vi "Periodic Tasks.vi"(8 "error in":errorcluster) -> ()   [LabVIEW 2018]
doc: "This VI runs in parallel to other tasks. It can contain as many user-defined periodic loops as you need. These can carry out PID or other sorts of timed response."
uses:
  <vilib>/Rock Robotics/WPI/Solenoid/WPI_SolenoidValue.ctl
  <vilib>/Rock Robotics/WPI/ThirdParty/Phoenix-LabVIEW/Motor Controller/Controls/CTRE_Phoenix_MotorControl_ControlMode.ctl
  <vilib>/Rock Robotics/WPI/DriverStation/WPI_DriverStationRobotMode2.ctl
  7c96cda5-b0e0-4e2a-8dae-2d02e7ea7fc2.vi
  ca579f97-49ab-43f2-8d57-79325bc44b91.vi
  49744297-d732-4f26-b9df-ea13e04ead65.vi
  0c7d2dc5-c582-4743-8fb3-b9c2bdc871ef.vi
  0ab41fdd-f005-4a41-8abb-d0c1aebc8839.vi
  eb1224c5-d191-4a5a-b208-f0176ff8254b.vi
  4d1e90e2-2e56-4cd0-9c54-8509fccd737b.vi
  fa0b2ed9-014b-4d02-a9e7-965de739ed34.vi
  3bc81077-0bee-49a4-9064-f6dc6ff34700.vi
  c6107473-3bbc-4d68-b130-33bb0f28684e.vi
  bc72f310-a025-467b-8a7d-9af20b832017.vi
  627df16c-e363-45ec-ab0c-cc0e3a3b33f7.vi
  ea05d6e2-4bc2-4863-96e4-0034388c650a.vi
  93672789-ce46-4bc6-a5b5-faff44e817a8.vi
  c8be7294-c6ee-427e-ae78-3199e8744a18.vi
  1c7609ed-6cb5-470b-bbb9-41d14296924d.vi
  50b6936b-a54e-4087-a151-83919d29fb22.vi
  efed0d96-a490-4904-9cbf-ad4873da1ad9.vi
  RobotStates.vi
  Robot Global Data.vi
  <vilib>/Rock Robotics/Network Tables/NT Write Number.vi
  RefNums_DriverStation.vi
  <vilib>/Rock Robotics/WPI/Utilities/WPI_GetSetVariantRefNum.vi
  RefNums_Actuators.vi
  <vilib>/Rock Robotics/WPI/Solenoid/WPI_SolenoidSetEnum.vi
  RefNums_Sensors.vi
  SensorReadings.vi
  Inputs_DriverStation.vi
panel:
  in  "Time in Error Band (ms)":u32=500
  in  "Error Band (in)":dbl=1.0
  in  "Max Down Power":dbl=-0.7 format="%#_13g"
  out "Sensor Loop (ms)":u32
  in  "Enable Plotting":bool
  out "Control Loop Time (ms)":u32
  out "PID Tracking":cluster{"Goal Wheel Position":dbl, dbl}(graph)={"Goal Wheel Position"=0.0, -90.17571233858979}
  out "Contribution Tracking":cluster{dbl, dbl, dbl}(graph)
  in  "N-Int":i32=25
  in  "N-Diff":i32=20
  in  "Kd":dbl=0.01
  in  "Ki":dbl=0.02
  in  "Kp":dbl=0.04
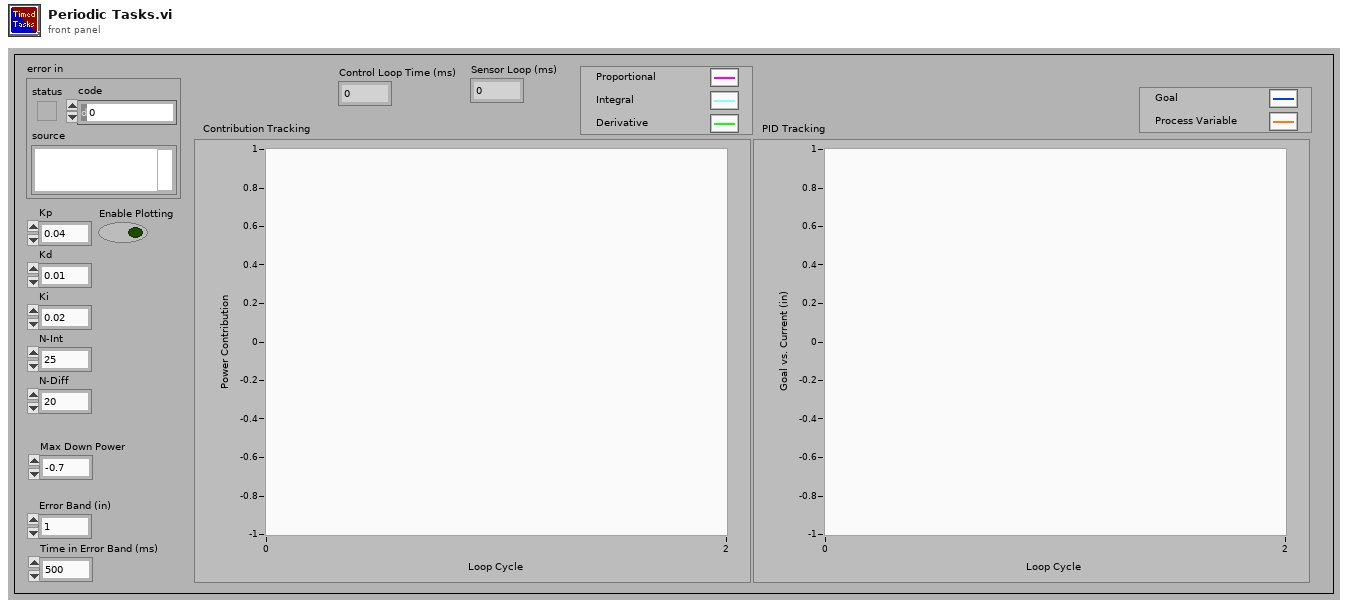
[diagram p1: front panel]
types:
  T1 = typedef "WPI_MotorControlDeviceRef.ctl" = cluster{"DeviceStatus":errorcluster, "Type":T2, "PWM":cluster{"PWM Channel":T3, "DeadBand":T4}, "CAN":cluster{"Device Number":u8, "SetOutput VI Ref":variant, "GetOutput VI Ref":variant, "Enable VI Ref":variant, "Disable VI Ref":variant, "Data":variant}, "Invert":bool, "DIO PWM":cluster{"PWM \"Enable\" Channel":T3, "DIOChannel":T5, "PWM Rate":dbl}}
  T2 = typedef "WPI_MotorControlType.ctl" = enum16{"PWM", "CAN", "DIO PWM"}
  T3 = typedef "FPGA_DIOPWMChannel.ctl" = enum8{"PWM 0", "PWM 1", "PWM 2", "PWM 3", "PWM 4", "PWM 5", "PWM 6", "PWM 7", "PWM 8", "PWM 9", "PWM MXP 0", "PWM MXP 1", "PWM MXP 2", "PWM MXP 3", "PWM MXP 4", "PWM MXP 5", "PWM MXP 6", "PWM MXP 7", "PWM MXP 8", "PWM MXP 9", "Invalid"}
  T4 = typedef "WPI_PWMDeadband.ctl" = cluster{"Name":string, "maxPositivePwm":i32, "minPositivePwm":i32, "centerPwm":i32, "maxNegativePwm":i32, "minNegativePwm":i32, "angularRange":u16}
  T5 = typedef "FPGA_DIOChannel.ctl" = enum8{"DIO 0", "DIO 1", "DIO 2", "DIO 3", "DIO 4", "DIO 5", "DIO 6", "DIO 7", "DIO 8", "DIO 9", "DIO MXP 0", "DIO MXP 1", "DIO MXP 2", "DIO MXP 3", "DIO MXP 4", "DIO MXP 5", "DIO MXP 6", "DIO MXP 7", "DIO MXP 8", "DIO MXP 9", "DIO MXP 10", "DIO MXP 11", "DIO MXP 12", "DIO MXP 13", "DIO MXP 14", "DIO MXP 15", "SPI Port CS1", "SPI Port CS2", "SPI Port CS3", "SPI Port MISO", "SPI Port MOSI", "Invalid"}
  T6 = typedef "WPI_SolenoidDevRef.ctl" = cluster{"DevStatus":errorcluster, "Pneumatics Control Module":u8, "Forward Solenoid Channel":T7, "Reverse Solenoid Channel":T7}
  T7 = typedef "WPI_SolenoidChannel.ctl" = enum8{"Solenoid 0", "Solenoid 1", "Solenoid 2", "Solenoid 3", "Solenoid 4", "Solenoid 5", "Solenoid 6", "Solenoid 7", "Invalid"}
  T8 = typedef "WPI_ServoDeviceRef.ctl" = cluster{"DeviceStatus":errorcluster, "PWM Channel":T3, "DeadBand":T4}
  T9 = typedef "WPI_JoystickDevRef.ctl" = cluster{"Device":T10}
  T10 = typedef "WPI_JoystickDeviceEnum.ctl" = enum16{"USB 0", "USB 1", "USB 2", "USB 3", "USB 4", "USB 5"}
  T11 = typedef "WPI_CompressorDevRef.ctl" = cluster{"DevStatus":errorcluster, "Pneumatics Control Module":u8}
  T12 = typedef "WPI_AccelerometerDevRef.ctl" = cluster{"DevStatus":errorcluster, "Scaling":T13, "Analog Channels":T14, "I2C Bus":T16, "SPI Bus":T17, "Accel Range":T18, "ADXL Axes":T19, "Handle":i32, "Device Address":u8, "Accel Type":enum16{"Analog", "ADXL345 I2C", "ADXL345 SPI", "Internal", "ADXL362 SPI"}}
  T13 = typedef "WPI_AccelerometerScaling.ctl" = cluster{"Gain (VoltsPerG)":dbl, "Center Voltage":dbl}
  T14 = typedef "WPI_AccelerometerAnalogChannels.ctl" = cluster{"X-Axis":T15, "Y-Axis":T15, "Z-Axis":T15}
  T15 = typedef "FPGA_AIChannel.ctl" = enum8{"AI 0", "AI 1", "AI 2", "AI 3", "AI MXP 0", "AI MXP 1", "AI MXP 2", "AI MXP 3", "Invalid"}
  T16 = typedef "i2c_bus.ctl" = enum16{"I2C On-Board", "I2C MXP", "Invalid"}
  T17 = typedef "spi_bus.ctl" = enum16{"SPI On-Board, CS0", "SPI On-Board, CS1", "SPI On-Board, CS2", "SPI On-Board, CS3", "SPI MXP", "Invalid"}
  T18 = typedef "ADXL345 Range.ctl" = u8
  T19 = typedef "WPI_AccelerometerADXL345 Axes.ctl" = cluster{"X-Axis":bool, "Y-Axis":bool, "Z-Axis":bool}
  T20 = typedef "WPI_AnalogChannelDevRef.ctl" = cluster{"DevStatus":errorcluster, "Analog Channel":T15}
  T21 = typedef "WPI_DriverStationRobotMode2.ctl" = enum16{"Autonomous Disabled", "Autonomous Enabled", "Teleop Disabled", "Teleop Enabled", "Disconnected", "Finish", "Test Disabled", "Test Enabled", "Emergency Stopped"}
  T22 = typedef "CTRE_Phoenix_MotorControl_ControlMode.ctl" = u16
  T23 = typedef "WPI_SolenoidValue.ctl" = enum16{"Off", "On", "Forward", "Reverse"}
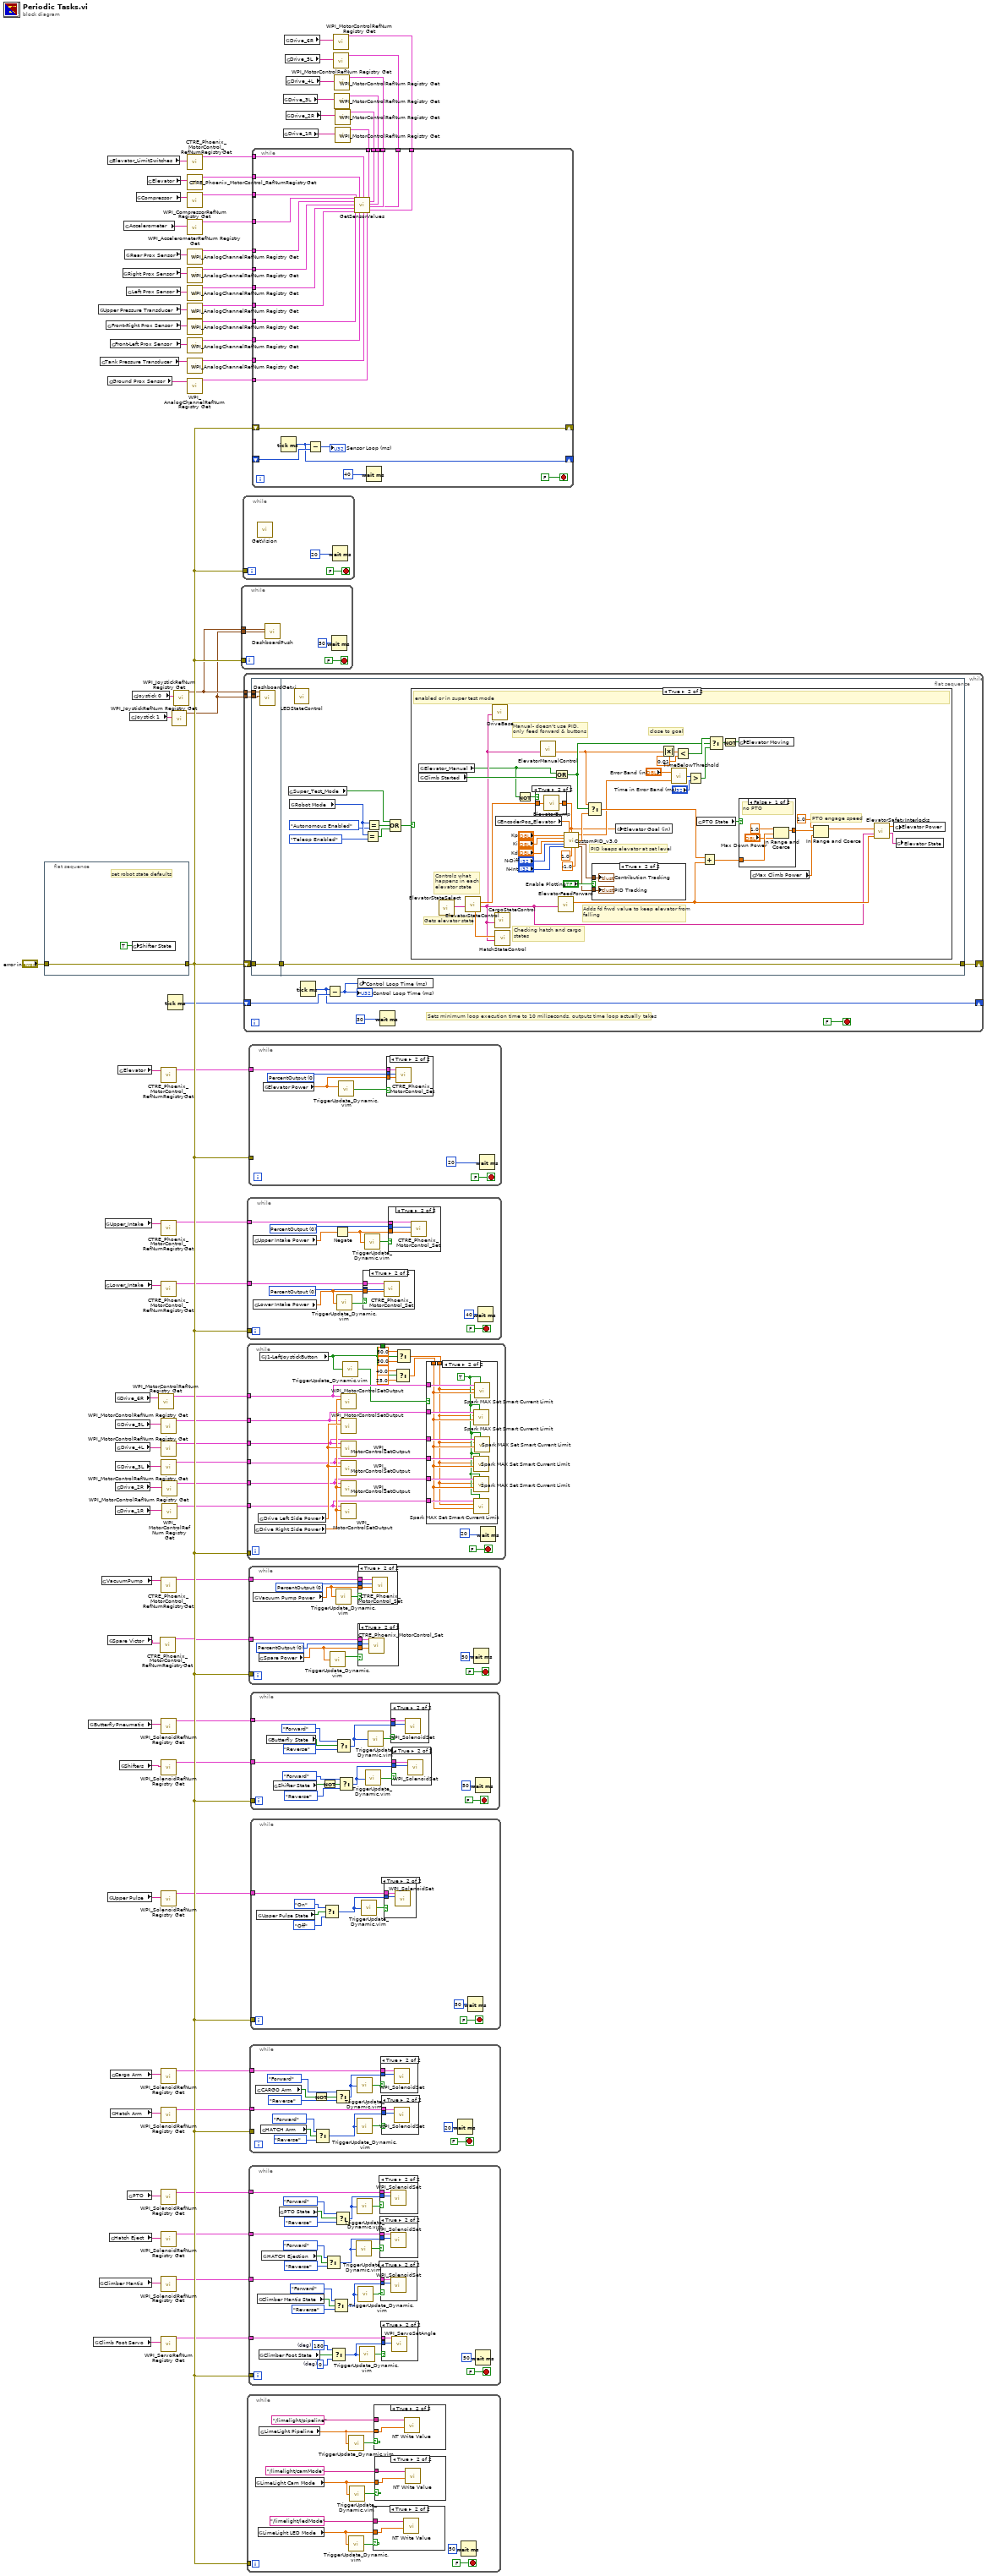
[diagram p0: block diagram]
diagram:
  n1 = flat-sequence {
    tunnel: [w85] -> w83
    tunnel: "error in" -> [w85]
    frame #0 {
      # "set robot state defaults"
      n2 = global write "RobotStates.vi" "Shifter State"(TRUE ("Shifter State")) -> ()
    }
  }
  n3 = global read "RefNums_Actuators.vi" "ButterflyPneumatic"() -> (w80:string)
  n4 = global read "RefNums_Actuators.vi" "Climb Foot Servo"() -> (w17:string)
  n5 = global read "RefNums_Sensors.vi" "Upper Pressure Transducer"() -> (w45:string)
  n6 = global read "RefNums_Actuators.vi" "Climber Mantis"() -> (w60:string)
  n7 = global read "RefNums_Sensors.vi" "Tank Pressure Transducer"() -> (w42:string)
  n8 = global read "RefNums_Actuators.vi" "VacuumPump"() -> (w73:string)
  n9 = global read "RefNums_Actuators.vi" "Upper_Intake"() -> (w70:string)
  n10 = global read "RefNums_Actuators.vi" "Lower_Intake"() -> (w69:string)
  n11 = global read "RefNums_Sensors.vi" "Front-Right Prox Sensor"() -> (w43:string)
  n12 = global read "RefNums_Actuators.vi" "Elevator_LimitSwitches"() -> (w31:string)
  n13 = global read "RefNums_Sensors.vi" "Ground Prox Sensor"() -> (w20:string)
  n14 = global read "RefNums_Actuators.vi" "Spare Victor"() -> (w66:string)
  n15 = global read "RefNums_Actuators.vi" "Upper Pulse"() -> (w76:string)
  n16 = global read "RefNums_Actuators.vi" "Hatch Eject"() -> (w61:string)
  n17 = global read "RefNums_Sensors.vi" "Front-Left Prox Sensor"() -> (w44:string)
  n18 = global read "RefNums_Actuators.vi" "Cargo Arm"() -> (w72:string)
  n19 = global read "RefNums_Actuators.vi" "Hatch Arm"() -> (w62:string)
  n20 = global read "RefNums_Actuators.vi" "Drive_6R"() -> (w14:string)
  n21 = global read "RefNums_Actuators.vi" "Drive_2R"() -> (w10:string)
  n22 = global read "RefNums_Actuators.vi" "Drive_1R"() -> (w15:string)
  n23 = global read "RefNums_Actuators.vi" "Drive_5L"() -> (w13:string)
  n24 = global read "RefNums_Actuators.vi" "Drive_4L"() -> (w12:string)
  n25 = global read "RefNums_Actuators.vi" "Drive_3L"() -> (w11:string)
  n26 = global read "RefNums_Actuators.vi" "Elevator"() -> (w36:string)
  n27 = global read "RefNums_Actuators.vi" "Shifters"() -> (w78:string)
  n28 = global read "RefNums_Sensors.vi" "Right Prox Sensor"() -> (w49:string)
  n29 = global read "RefNums_Sensors.vi" "Accelerometer"() -> (w23:string)
  n30 = global read "RefNums_Sensors.vi" "Rear Prox Sensor"() -> (w51:string)
  n31 = global read "RefNums_Sensors.vi" "Left Prox Sensor"() -> (w50:string)
  n32 = global read "RefNums_Actuators.vi" "PTO"() -> (w64:string)
  n33 = global read "RefNums_DriverStation.vi" "Joystick 1"() -> (w35:string)
  n34 = global read "RefNums_DriverStation.vi" "Joystick 0"() -> (w81:string)
  n35 = global read "RefNums_Actuators.vi" "Compressor"() -> (w55:string)
  n36 = global read "RefNums_Actuators.vi" "Elevator"() -> (w54:string)
  n37 = call <vilib>:"WPI_MotorControlRefNum Registry Get.vi"("refnum name"=w14) -> ("MotorControlDevRef"=w5:T1)  [unwired: 9 in, 1 out]
  n38 = call <vilib>:"CTRE_Phoenix_MotorControl_RefNumRegistryGet.vi"("refnum name"=w66) -> ("PhoenixMotorControlDevRef"=w65:T1)  [unwired: 9 in, 1 out]
  n39 = call <vilib>:"CTRE_Phoenix_MotorControl_RefNumRegistryGet.vi"("refnum name"=w36) -> ("PhoenixMotorControlDevRef"=w82:T1)  [unwired: 9 in, 1 out]
  n40 = call <vilib>:"CTRE_Phoenix_MotorControl_RefNumRegistryGet.vi"("refnum name"=w70) -> ("PhoenixMotorControlDevRef"=w68:T1)  [unwired: 9 in, 1 out]
  n41 = call <vilib>:"CTRE_Phoenix_MotorControl_RefNumRegistryGet.vi"("refnum name"=w69) -> ("PhoenixMotorControlDevRef"=w67:T1)  [unwired: 9 in, 1 out]
  n42 = call <vilib>:"CTRE_Phoenix_MotorControl_RefNumRegistryGet.vi"("refnum name"=w73) -> ("PhoenixMotorControlDevRef"=w74:T1)  [unwired: 9 in, 1 out]
  n43 = call <vilib>:"WPI_SolenoidRefNum Registry Get.vi"("refnum name"=w80) -> ("SolenoidDevRef"=w79:T6)  [unwired: 9 in, 1 out]
  n44 = call <vilib>:"WPI_SolenoidRefNum Registry Get.vi"("refnum name"=w78) -> ("SolenoidDevRef"=w77:T6)  [unwired: 9 in, 1 out]
  n45 = call <vilib>:"WPI_SolenoidRefNum Registry Get.vi"("refnum name"=w76) -> ("SolenoidDevRef"=w75:T6)  [unwired: 9 in, 1 out]
  n46 = call <vilib>:"WPI_SolenoidRefNum Registry Get.vi"("refnum name"=w72) -> ("SolenoidDevRef"=w71:T6)  [unwired: 9 in, 1 out]
  n47 = call <vilib>:"WPI_SolenoidRefNum Registry Get.vi"("refnum name"=w62) -> ("SolenoidDevRef"=w59:T6)  [unwired: 9 in, 1 out]
  n48 = call <vilib>:"WPI_SolenoidRefNum Registry Get.vi"("refnum name"=w64) -> ("SolenoidDevRef"=w63:T6)  [unwired: 9 in, 1 out]
  n49 = call <vilib>:"WPI_SolenoidRefNum Registry Get.vi"("refnum name"=w61) -> ("SolenoidDevRef"=w58:T6)  [unwired: 9 in, 1 out]
  n50 = call <vilib>:"WPI_SolenoidRefNum Registry Get.vi"("refnum name"=w60) -> ("SolenoidDevRef"=w57:T6)  [unwired: 9 in, 1 out]
  n51 = call <vilib>:"WPI_ServoRefNum Registry Get.vi"("refnum name"=w17) -> ("ServoDeviceRef"=w18:T8)  [unwired: 9 in, 1 out]
  n52 = call <vilib>:"WPI_MotorControlRefNum Registry Get.vi"("refnum name"=w13) -> ("MotorControlDevRef"=w6:T1)  [unwired: 9 in, 1 out]
  n53 = call <vilib>:"WPI_MotorControlRefNum Registry Get.vi"("refnum name"=w12) -> ("MotorControlDevRef"=w7:T1)  [unwired: 9 in, 1 out]
  n54 = call <vilib>:"WPI_MotorControlRefNum Registry Get.vi"("refnum name"=w11) -> ("MotorControlDevRef"=w8:T1)  [unwired: 9 in, 1 out]
  n55 = call <vilib>:"WPI_MotorControlRefNum Registry Get.vi"("refnum name"=w10) -> ("MotorControlDevRef"=w9:T1)  [unwired: 9 in, 1 out]
  n56 = call <vilib>:"WPI_MotorControlRefNum Registry Get.vi"("refnum name"=w15) -> ("MotorControlDevRef"=w16:T1)  [unwired: 9 in, 1 out]
  n57 = Tick Count (ms)() -> (millisecond timer value=w56:u32)
  n58 = call <vilib>:"WPI_JoystickRefNum Registry Get.vi"("refnum name"=w35) -> ("JoystickDevRef"=w21:T9)  [unwired: 9 in, 1 out]
  n59 = call <vilib>:"WPI_JoystickRefNum Registry Get.vi"("refnum name"=w81) -> ("JoystickDevRef"=w37:T9)  [unwired: 9 in, 1 out]
  n60 = call <vilib>:"CTRE_Phoenix_MotorControl_RefNumRegistryGet.vi"("refnum name"=w31) -> ("PhoenixMotorControlDevRef"=w30:T1)  [unwired: 9 in, 1 out]
  n61 = call <vilib>:"CTRE_Phoenix_MotorControl_RefNumRegistryGet.vi"("refnum name"=w54) -> ("PhoenixMotorControlDevRef"=w53:T1)  [unwired: 9 in, 1 out]
  n62 = call <vilib>:"WPI_CompressorRefNum Registry Get.vi"("refnum name"=w55) -> ("CompressorDevRef"=w52:T11)  [unwired: 9 in, 1 out]
  n63 = call <vilib>:"WPI_AccelerometerRefNum Registry Get.vi"("refnum name"=w23) -> ("AccelerometerDevRef"=w22:T12)  [unwired: 9 in, 1 out]
  n64 = call <vilib>:"WPI_AnalogChannelRefNum Registry Get.vi"("refnum name"=w51) -> ("AIDeviceRef"=w48:T20)  [unwired: 9 in, 1 out]
  n65 = call <vilib>:"WPI_AnalogChannelRefNum Registry Get.vi"("refnum name"=w49) -> ("AIDeviceRef"=w47:T20)  [unwired: 9 in, 1 out]
  n66 = call <vilib>:"WPI_AnalogChannelRefNum Registry Get.vi"("refnum name"=w50) -> ("AIDeviceRef"=w46:T20)  [unwired: 9 in, 1 out]
  n67 = call <vilib>:"WPI_AnalogChannelRefNum Registry Get.vi"("refnum name"=w45) -> ("AIDeviceRef"=w41:T20)  [unwired: 9 in, 1 out]
  n68 = call <vilib>:"WPI_AnalogChannelRefNum Registry Get.vi"("refnum name"=w43) -> ("AIDeviceRef"=w40:T20)  [unwired: 9 in, 1 out]
  n69 = call <vilib>:"WPI_AnalogChannelRefNum Registry Get.vi"("refnum name"=w44) -> ("AIDeviceRef"=w39:T20)  [unwired: 9 in, 1 out]
  n70 = call <vilib>:"WPI_AnalogChannelRefNum Registry Get.vi"("refnum name"=w42) -> ("AIDeviceRef"=w38:T20)  [unwired: 9 in, 1 out]
  n71 = call <vilib>:"WPI_AnalogChannelRefNum Registry Get.vi"("refnum name"=w20) -> ("AIDeviceRef"=w19:T20)  [unwired: 9 in, 1 out]
  n72 = while {
    tunnel: w37 -> [w88]
    tunnel: w83 -> [_]
    tunnel: w21 -> [w86]
    stop <- FALSE stop-if-true
    n73 = call "DashboardPush.vi"("Joystick 0 Ref"=w88, "Joystick 1 Ref"=w86) -> ()  [unwired: 14 in]
    n74 = Wait (ms)(milliseconds to wait=u32 50) -> ()  [unwired: 1 out]
  }
  n75 = while {
    tunnel: w83 -> [_]
    stop <- FALSE stop-if-true
    n76 = call "GetVision.vi"() -> ()  [unwired: 12 in]
    n77 = Wait (ms)(milliseconds to wait=u32 20) -> ()  [unwired: 1 out]
  }
  n78 = while {
    shift-right: [w98] -> _
    shift-left: w83 -> [w100]
    tunnel: w37 -> [w97]
    shift-right: [w95] -> _
    shift-left: w56 -> [w96]
    tunnel: w21 -> [w93]
    stop <- FALSE stop-if-true
    # "Sets minimum loop execution time to 10 miliseconds, outputs time loop actually takes"
    n79 = flat-sequence {
      tunnel: w97 -> [w104]
      tunnel: w100 -> [w103]
      tunnel: [w103] -> w99
      tunnel: w93 -> [w102]
      tunnel: w99 -> [w112]
      tunnel: [w112] -> w98
      frame #0 {
        n80 = call "DashboardGetvi.vi"("Joystick 2"=w102, "Joystick 1"=w104) -> ()  [unwired: 8 in]
      }
      frame #1 {
        n81 = global read "Inputs_DriverStation.vi" "Super_Test_Mode"() -> (w105:bool)
        n82 = global read "Robot Global Data.vi" "Robot Mode"() -> (w109:T21)
        n83 = call "LEDStateControl.vi"() -> ()  [unwired: 12 in]
        n84 = Equal?(x=w109, y=WPI_DriverStationRobotMode2."Teleop Enabled") -> (x = y?=w110:bool)
        n85 = Equal?(x=w109, y=WPI_DriverStationRobotMode2."Autonomous Enabled") -> (x = y?=w111:bool)
        n86 = Compound Arithmetic op=OR(w105, w111, w110) -> (w106:bool)
        n87 = case shown="True" w106 {
          frame False {
            # "disabled and not in super test mode"
          }
          frame True {
            # "PTO engage speed"
            # "close to goal"
            # "PID keeps elevator at set level"
            # "Manual- doesn't use PID,\nonly feed forward & buttons"
            # "Adds fd frwd value to keep elevator from falling"
            # "Checking hatch and cargo \nstates"
            # "Controls what\nhappens in each \nelevator state"
            # "Gets elevator state"
            # "enabled or in super test mode"
            n88 = global read "Inputs_DriverStation.vi" "Elevator_Manual"() -> (w113:bool)
            n89 = global read "RobotStates.vi" "Climb Started"() -> (w138:bool)
            n90 = call "ElevatorStateSelect.vi"() -> ("Elevator State"=w151:string)  [unwired: 11 in]
            n91 = call "ElevatorStateControl.vi"("Elevator State"=w151) -> ("Elevator State Out"=w121:string, "Target Elevator Position"=w154:dbl, "Target Vacuum Pump Power"=w139:dbl)  [unwired: 8 in]
            n92 = call "DriveBase.vi"("Elevator State"=w121) -> ()  [unwired: 11 in]
            n93 = call "CargoStateControl.vi"("Elevator State"=w121) -> ()  [unwired: 11 in]
            n94 = call "HatchStateControl.vi"("Elevator State"=w121, "Vacuum Pump Power"=w139) -> ()  [unwired: 10 in]
            n95 = global read "SensorReadings.vi" "EncoderPos_Elevator"() -> (w149:dbl)
            n96 = Not(x=w113) -> (.not. x?=w114:bool)
            n97 = case shown="True" w114 {
              tunnel: w154 -> [w155 w157]
              tunnel: [w155 w156] -> w115
              frame False {
              }
              frame True {
                n98 = call "ElevatorBump.vi"("Elevator Goal In (in)"=w157) -> ("Elevator Goal Out (in)"=w156:dbl)
              }
            }
            n99 = call "ElevatorManualControl.vi"("Elevator State"=w121) -> ("Manual Contribution"=w122:dbl)  [unwired: 10 in]
            n100 = Or(x=w113, y=w138) -> (x .or. y?=w124:bool)
            n101 = call "ElevatorFeedForward.vi"("Elevator State"=w121) -> ("Feed Forward Contribution"=w135:dbl)  [unwired: 10 in]
            n102 = call "CustomPID_v3.0.vi"("Kp"="Kp", "Process Variable"=w149, "Goal"=w115, "Ki"="Ki", "Kd"="Kd", "N-Diff"="N-Diff", "N-Int"="N-Int", "Max Ouput"=1.0, "Min Output"=-1.0) -> ("Current Error"=w130:dbl, "Command"=w150:dbl, "Contribution Tracking"=w141:cluster{dbl, dbl, dbl}, "PID Tracking"=w140:cluster{"Goal Wheel Position":dbl, dbl})  [unwired: 3 in]
            n103 = Select(t=w122, s=w124, f=w150) -> (s? t:f=w152:dbl)
            n104 = case shown="True" "Enable Plotting" {
              tunnel: w141 -> [_ w167]
              tunnel: w140 -> [_ w166]
              frame False {
              }
              frame True {
                "Contribution Tracking" <- w167
                "PID Tracking" <- w166
              }
            }
            n105 = global write "RobotStates.vi" "Elevator Goal (in)"(w115) -> ()
            n106 = Absolute Value(x=w122) -> (abs(x)=w129:dbl)
            n107 = call "TimeBelowThreshold.vi"("Current Value"=w130, "Threshold"="Error Band (in)") -> ("Time Below"=w132:u32)  [unwired: 3 in]
            n108 = Less?(x=w129, y=0.01) -> (x < y?=w128:bool)
            n109 = Greater?(x=w132, y="Time in Error Band (ms)") -> (0:w123:bool)
            n110 = global read "RobotStates.vi" "PTO State"() -> (w120:bool)
            n111 = Add(x=w152, y=w135) -> (x+y=w134:dbl)
            n112 = Select(t=w128, s=w124, f=w123) -> (s? t:f=w127:bool)
            n113 = Not(x=w127) -> (.not. x?=w126:bool)
            n114 = global write "RobotStates.vi" "Elevator Moving"(w126) -> ()
            n115 = case shown="False" w120 {
              tunnel: w134 -> [w161 w164]
              tunnel: [w158 w165] -> w118
              frame False {
                # "no PTO"
                n116 = In Range and Coerce(upper limit=1.0, x=w161, lower limit="Max Down Power") -> (coerced(x)=w158:dbl)  [unwired: 1 out]
              }
              frame True {
                # "PTO"
                n117 = In Range and Coerce(upper limit=1.0, x=w164, lower limit=-1.0) -> (coerced(x)=w165:dbl)  [unwired: 1 out]
              }
            }
            n118 = global read "RobotStates.vi" "Max Climb Power"() -> (w116:dbl)
            n119 = In Range and Coerce(upper limit=1.0, x=w118, lower limit=w116) -> (coerced(x)=w119:dbl)  [unwired: 1 out]
            n120 = call "ElevatorSafetyInterlocks.vi"("Feed Forward Contribution"=w135, "Elevator State In"=w121, "Elevator Power In"=w119) -> ("Elevator State Out"=w136:string, "Elevator Power Out"=w137:dbl)  [unwired: 7 in]
            n121 = global write "RobotStates.vi" "Elevator Power"(w137) -> ()
            n122 = global write "RobotStates.vi" "Elevator State"(w136) -> ()
          }
        }
      }
    }
    n123 = Tick Count (ms)() -> (millisecond timer value=w95:u32)
    n124 = Subtract(x=w95, y=w96) -> (x-y=w94:u32)
    "Control Loop Time (ms)" <- w94
    n125 = global write "SensorReadings.vi" "Control Loop Time (ms)"(w94) -> ()
    n126 = Wait (ms)(milliseconds to wait=u32 30) -> ()  [unwired: 1 out]
  }
  n127 = while {
    tunnel: w83 -> [_]
    tunnel: w16 -> [w181]
    tunnel: w9 -> [w180]
    tunnel: w8 -> [w179]
    tunnel: w7 -> [w178]
    tunnel: w6 -> [w177]
    tunnel: w5 -> [w176]
    tunnel: [w168] -> _
    stop <- FALSE stop-if-true
    n128 = global read "RobotStates.vi" "Drive Right Side Power"() -> (w182:dbl)
    n129 = global read "RobotStates.vi" "Drive Left Side Power"() -> (w183:dbl)
    n130 = global read "Inputs_DriverStation.vi" "J1-LeftJoystickButton"() -> (w168:bool)
    n131 = call <vilib>:"WPI_MotorControlSetOutput.vi"("Output"=w182, "MotorControlDevRef"=w176) -> ()  [unwired: 7 in, 3 out]
    n132 = call <vilib>:"WPI_MotorControlSetOutput.vi"("Output"=w183, "MotorControlDevRef"=w177) -> ()  [unwired: 7 in, 3 out]
    n133 = call <vilib>:"WPI_MotorControlSetOutput.vi"("Output"=w183, "MotorControlDevRef"=w178) -> ()  [unwired: 7 in, 3 out]
    n134 = call <vilib>:"WPI_MotorControlSetOutput.vi"("Output"=w183, "MotorControlDevRef"=w179) -> ()  [unwired: 7 in, 3 out]
    n135 = call <vilib>:"WPI_MotorControlSetOutput.vi"("Output"=w182, "MotorControlDevRef"=w180) -> ()  [unwired: 7 in, 3 out]
    n136 = call <vilib>:"WPI_MotorControlSetOutput.vi"("Output"=w182, "MotorControlDevRef"=w181) -> ()  [unwired: 7 in, 3 out]
    n137 = call "TriggerUpdate_Dynamic.vim"("Trigger"=w168) -> ("Update"=w169:bool)
    n138 = Select(t=40.0, s=w168, f=25.0 ("Free Speed Current Limit (20A)")) -> (s? t:f=w174:dbl)
    n139 = Select(t=80.0, s=w168, f=50.0 ("Free Speed Current Limit (20A)")) -> (s? t:f=w170:dbl)
    n140 = case shown="True" w169 {
      tunnel: w181 -> [_ w194]
      tunnel: w180 -> [_ w193]
      tunnel: w179 -> [_ w192]
      tunnel: w178 -> [_ w191]
      tunnel: w177 -> [_ w190]
      tunnel: w176 -> [_ w189]
      tunnel: w174 -> [_ w188]
      tunnel: w170 -> [_ w186]
      frame False {
      }
      frame True {
        w187 = TRUE
        n141 = call <vilib>:"Spark MAX Set Smart Current Limit.vi"("Linearized Limit Enabled (F)"=w187, "Free Speed Current Limit (20A)"=w188, "Primay Current Limit (80A)"=w186, "MotorControlDeviceRef in"=w192) -> ()  [unwired: 6 in, 2 out]
        n142 = call <vilib>:"Spark MAX Set Smart Current Limit.vi"("Linearized Limit Enabled (F)"=w187, "Free Speed Current Limit (20A)"=w188, "Primay Current Limit (80A)"=w186, "MotorControlDeviceRef in"=w190) -> ()  [unwired: 6 in, 2 out]
        n143 = call <vilib>:"Spark MAX Set Smart Current Limit.vi"("Linearized Limit Enabled (F)"=w187, "Free Speed Current Limit (20A)"=w188, "Primay Current Limit (80A)"=w186, "MotorControlDeviceRef in"=w193) -> ()  [unwired: 6 in, 2 out]
        n144 = call <vilib>:"Spark MAX Set Smart Current Limit.vi"("Linearized Limit Enabled (F)"=w187, "Free Speed Current Limit (20A)"=w188, "Primay Current Limit (80A)"=w186, "MotorControlDeviceRef in"=w194) -> ()  [unwired: 6 in, 2 out]
        n145 = call <vilib>:"Spark MAX Set Smart Current Limit.vi"("Linearized Limit Enabled (F)"=w187, "Free Speed Current Limit (20A)"=w188, "Primay Current Limit (80A)"=w186, "MotorControlDeviceRef in"=w189) -> ()  [unwired: 6 in, 2 out]
        n146 = call <vilib>:"Spark MAX Set Smart Current Limit.vi"("Linearized Limit Enabled (F)"=w187, "Free Speed Current Limit (20A)"=w188, "Primay Current Limit (80A)"=w186, "MotorControlDeviceRef in"=w191) -> ()  [unwired: 6 in, 2 out]
      }
    }
    n147 = Wait (ms)(milliseconds to wait=u32 20) -> ()  [unwired: 1 out]
  }
  n148 = while {
    tunnel: w83 -> [_]
    stop <- FALSE stop-if-true
    n149 = global read "RobotStates.vi" "LimeLight Cam Mode"() -> (w198:dbl)
    n150 = global read "RobotStates.vi" "LimeLight LED Mode"() -> (w201:dbl)
    n151 = global read "RobotStates.vi" "LimeLight Pipeline"() -> (w195:dbl)
    n152 = call "TriggerUpdate_Dynamic.vim"("Trigger"=w201) -> ("Update"=w203:bool)
    n153 = call "TriggerUpdate_Dynamic.vim"("Trigger"=w195) -> ("Update"=w197:bool)
    n154 = call "TriggerUpdate_Dynamic.vim"("Trigger"=w198) -> ("Update"=w200:bool)
    n155 = case shown="True" w203 {
      tunnel: "/limelight/ledMode" ("Name") -> [_ w211]
      tunnel: w201 -> [_ w210]
      frame False {
      }
      frame True {
        n156 = call-poly <vilib>:"NT Write Value.vi"("Numeric"=w210, "Name"=w211) -> ()  [unwired: 9 in, 1 out]
      }
    }
    n157 = case shown="True" w197 {
      tunnel: "/limelight/pipeline" ("Name") -> [_ w207]
      tunnel: w195 -> [_ w206]
      frame False {
      }
      frame True {
        n158 = call-poly <vilib>:"NT Write Value.vi"("Numeric"=w206, "Name"=w207) -> ()  [unwired: 9 in, 1 out]
      }
    }
    n159 = case shown="True" w200 {
      tunnel: "/limelight/camMode" ("Name") -> [_ w209]
      tunnel: w198 -> [_ w208]
      frame False {
      }
      frame True {
        n160 = call-poly <vilib>:"NT Write Value.vi"("Numeric"=w208, "Name"=w209) -> ()  [unwired: 9 in, 1 out]
      }
    }
    n161 = Wait (ms)(milliseconds to wait=u32 50) -> ()  [unwired: 1 out]
  }
  n162 = while {
    tunnel: w68 -> [w222]
    tunnel: w67 -> [w221]
    tunnel: w83 -> [_]
    stop <- FALSE stop-if-true
    w219 = T22 0 items=["PercentOutput"=0, "Position"=1, "Velocity"=2, "Current"=3, "Follower"=5, "MotionProfile"=6, "MotionMagic"=7, "MotionProfileArc"=10, "Disabled"=15] ("Control Mode")
    w220 = T22 0 items=["PercentOutput"=0, "Position"=1, "Velocity"=2, "Current"=3, "Follower"=5, "MotionProfile"=6, "MotionMagic"=7, "MotionProfileArc"=10, "Disabled"=15] ("Control Mode")
    n163 = global read "RobotStates.vi" "Upper Intake Power"() -> (w216:dbl)
    n164 = global read "RobotStates.vi" "Lower Intake Power"() -> (w214:dbl)
    n165 = Negate(x=w216) -> (-x=w212:dbl)
    n166 = call "TriggerUpdate_Dynamic.vim"("Trigger"=w214) -> ("Update"=w213:bool)
    n167 = case shown="True" w213 {
      tunnel: w221 -> [_ w225]
      tunnel: w219 -> [_ w224]
      tunnel: w214 -> [_ w223]
      frame False {
      }
      frame True {
        n168 = call <vilib>:"CTRE_Phoenix_MotorControl_Set.vi"("Output"=w223, "Control Mode"=w224, "PhoenixMotorControlDevRef"=w225) -> ()  [unwired: 7 in, 2 out]
      }
    }
    n169 = call "TriggerUpdate_Dynamic.vim"("Trigger"=w212) -> ("Update"=w215:bool)
    n170 = case shown="True" w215 {
      tunnel: w222 -> [_ w228]
      tunnel: w220 -> [_ w227]
      tunnel: w212 -> [_ w226]
      frame False {
      }
      frame True {
        n171 = call <vilib>:"CTRE_Phoenix_MotorControl_Set.vi"("Output"=w226, "Control Mode"=w227, "PhoenixMotorControlDevRef"=w228) -> ()  [unwired: 7 in, 2 out]
      }
    }
    n172 = Wait (ms)(milliseconds to wait=u32 40) -> ()  [unwired: 1 out]
  }
  n173 = while {
    tunnel: w83 -> [_]
    tunnel: w82 -> [w233]
    stop <- FALSE stop-if-true
    w232 = T22 0 items=["PercentOutput"=0, "Position"=1, "Velocity"=2, "Current"=3, "Follower"=5, "MotionProfile"=6, "MotionMagic"=7, "MotionProfileArc"=10, "Disabled"=15] ("Control Mode")
    n174 = global read "RobotStates.vi" "Elevator Power"() -> (w231:dbl)
    n175 = call "TriggerUpdate_Dynamic.vim"("Trigger"=w231) -> ("Update"=w230:bool)
    n176 = case shown="True" w230 {
      tunnel: w233 -> [_ w237]
      tunnel: w232 -> [_ w236]
      tunnel: w231 -> [_ w235]
      frame False {
      }
      frame True {
        n177 = call <vilib>:"CTRE_Phoenix_MotorControl_Set.vi"("Output"=w235, "Control Mode"=w236, "PhoenixMotorControlDevRef"=w237) -> ()  [unwired: 7 in, 2 out]
      }
    }
    n178 = Wait (ms)(milliseconds to wait=u32 20) -> ()  [unwired: 1 out]
  }
  n179 = while {
    tunnel: w74 -> [w247]
    tunnel: w65 -> [w246]
    tunnel: w83 -> [_]
    stop <- FALSE stop-if-true
    w238 = T22 0 items=["PercentOutput"=0, "Position"=1, "Velocity"=2, "Current"=3, "Follower"=5, "MotionProfile"=6, "MotionMagic"=7, "MotionProfileArc"=10, "Disabled"=15] ("Control Mode")
    w245 = T22 0 items=["PercentOutput"=0, "Position"=1, "Velocity"=2, "Current"=3, "Follower"=5, "MotionProfile"=6, "MotionMagic"=7, "MotionProfileArc"=10, "Disabled"=15] ("Control Mode")
    n180 = global read "RobotStates.vi" "Vacuum Pump Power"() -> (w242:dbl)
    n181 = global read "RobotStates.vi" "Spare Power"() -> (w240:dbl)
    n182 = call "TriggerUpdate_Dynamic.vim"("Trigger"=w240) -> ("Update"=w239:bool)
    n183 = call "TriggerUpdate_Dynamic.vim"("Trigger"=w242) -> ("Update"=w241:bool)
    n184 = case shown="True" w241 {
      tunnel: w247 -> [_ w253]
      tunnel: w245 -> [_ w252]
      tunnel: w242 -> [_ w251]
      frame False {
      }
      frame True {
        n185 = call <vilib>:"CTRE_Phoenix_MotorControl_Set.vi"("Output"=w251, "Control Mode"=w252, "PhoenixMotorControlDevRef"=w253) -> ()  [unwired: 7 in, 2 out]
      }
    }
    n186 = case shown="True" w239 {
      tunnel: w246 -> [_ w250]
      tunnel: w238 -> [_ w249]
      tunnel: w240 -> [_ w248]
      frame False {
      }
      frame True {
        n187 = call <vilib>:"CTRE_Phoenix_MotorControl_Set.vi"("Output"=w248, "Control Mode"=w249, "PhoenixMotorControlDevRef"=w250) -> ()  [unwired: 7 in, 2 out]
      }
    }
    n188 = Wait (ms)(milliseconds to wait=u32 50) -> ()  [unwired: 1 out]
  }
  n189 = while {
    tunnel: w63 -> [w279]
    tunnel: w58 -> [w278]
    tunnel: w57 -> [w277]
    tunnel: w83 -> [_]
    tunnel: w18 -> [w258]
    stop <- FALSE stop-if-true
    w255 = 180  # (deg)
    w257 = 0  # (deg)
    n190 = global read "RobotStates.vi" "Climber Mantis State"() -> (w272:bool)
    n191 = global read "RobotStates.vi" "Climber Foot State"() -> (w254:bool)
    n192 = global read "RobotStates.vi" "HATCH Ejection"() -> (w274:bool)
    n193 = global read "RobotStates.vi" "PTO State"() -> (w260:bool)
    n194 = Select(t=WPI_SolenoidValue."Forward" ("Value"), s=w274, f=WPI_SolenoidValue."Reverse") -> (s? t:f=w264:T23)
    n195 = Select(t=w255, s=w254, f=w257) -> (s? t:f=w256:i32)
    n196 = Select(t=WPI_SolenoidValue."Forward" ("Value"), s=w272, f=WPI_SolenoidValue."Reverse") -> (s? t:f=w262:T23)
    n197 = Select(t=WPI_SolenoidValue."Forward" ("Value"), s=w260, f=WPI_SolenoidValue."Reverse") -> (s? t:f=w266:T23)
    n198 = call "TriggerUpdate_Dynamic.vim"("Trigger"=w264) -> ("Update"=w263:bool)
    n199 = call "TriggerUpdate_Dynamic.vim"("Trigger"=w266) -> ("Update"=w265:bool)
    n200 = call "TriggerUpdate_Dynamic.vim"("Trigger"=w262) -> ("Update"=w261:bool)
    n201 = call "TriggerUpdate_Dynamic.vim"("Trigger"=w256) -> ("Update"=w259:bool)
    n202 = case shown="True" w265 {
      tunnel: w279 -> [_ w287]
      tunnel: w266 -> [_ w286]
      frame False {
      }
      frame True {
        n203 = call-poly <vilib>:"WPI_SolenoidSet.vi"("Value"=w286, "SolenoidDevRef"=w287) -> ()  [unwired: 8 in, 2 out]
      }
    }
    n204 = case shown="True" w263 {
      tunnel: w278 -> [_ w285]
      tunnel: w264 -> [_ w284]
      frame False {
      }
      frame True {
        n205 = call-poly <vilib>:"WPI_SolenoidSet.vi"("Value"=w284, "SolenoidDevRef"=w285) -> ()  [unwired: 8 in, 2 out]
      }
    }
    n206 = case shown="True" w261 {
      tunnel: w277 -> [_ w283]
      tunnel: w262 -> [_ w282]
      frame False {
      }
      frame True {
        n207 = call-poly <vilib>:"WPI_SolenoidSet.vi"("Value"=w282, "SolenoidDevRef"=w283) -> ()  [unwired: 8 in, 2 out]
      }
    }
    n208 = case shown="True" w259 {
      tunnel: w256 -> [_ w280]
      tunnel: w258 -> [_ w281]
      frame False {
      }
      frame True {
        n209 = call <vilib>:"WPI_ServoSetAngle.vi"("Angle"=w280, "ServoDeviceRef"=w281) -> ()  [unwired: 8 in, 2 out]
      }
    }
    n210 = Wait (ms)(milliseconds to wait=u32 50) -> ()  [unwired: 1 out]
  }
  n211 = while {
    tunnel: w71 -> [w302]
    tunnel: w59 -> [w301]
    tunnel: w83 -> [_]
    stop <- FALSE stop-if-true
    n212 = global read "RobotStates.vi" "CARGO Arm"() -> (w300:bool)
    n213 = global read "RobotStates.vi" "HATCH Arm"() -> (w297:bool)
    n214 = Not(x=w300) -> (.not. x?=w288:bool)
    n215 = Select(t=WPI_SolenoidValue."Forward" ("Value"), s=w297, f=WPI_SolenoidValue."Reverse") -> (s? t:f=w290:T23)
    n216 = Select(t=WPI_SolenoidValue."Forward" ("Value"), s=w288, f=WPI_SolenoidValue."Reverse") -> (s? t:f=w292:T23)
    n217 = call "TriggerUpdate_Dynamic.vim"("Trigger"=w292) -> ("Update"=w291:bool)
    n218 = call "TriggerUpdate_Dynamic.vim"("Trigger"=w290) -> ("Update"=w289:bool)
    n219 = case shown="True" w291 {
      tunnel: w302 -> [_ w306]
      tunnel: w292 -> [_ w305]
      frame False {
      }
      frame True {
        n220 = call-poly <vilib>:"WPI_SolenoidSet.vi"("Value"=w305, "SolenoidDevRef"=w306) -> ()  [unwired: 8 in, 2 out]
      }
    }
    n221 = case shown="True" w289 {
      tunnel: w301 -> [_ w304]
      tunnel: w290 -> [_ w303]
      frame False {
      }
      frame True {
        n222 = call-poly <vilib>:"WPI_SolenoidSet.vi"("Value"=w303, "SolenoidDevRef"=w304) -> ()  [unwired: 8 in, 2 out]
      }
    }
    n223 = Wait (ms)(milliseconds to wait=u32 20) -> ()  [unwired: 1 out]
  }
  n224 = while {
    tunnel: w79 -> [w321]
    tunnel: w77 -> [w320]
    tunnel: w83 -> [_]
    stop <- FALSE stop-if-true
    n225 = global read "RobotStates.vi" "Butterfly State"() -> (w317:bool)
    n226 = global read "RobotStates.vi" "Shifter State"() -> (w316:bool)
    n227 = Not(x=w316) -> (.not. x?=w307:bool)
    n228 = Select(t=WPI_SolenoidValue."Forward" ("Value"), s=w317, f=WPI_SolenoidValue."Reverse") -> (s? t:f=w311:T23)
    n229 = Select(t=WPI_SolenoidValue."Forward" ("Value"), s=w307, f=WPI_SolenoidValue."Reverse") -> (s? t:f=w309:T23)
    n230 = call "TriggerUpdate_Dynamic.vim"("Trigger"=w309) -> ("Update"=w308:bool)
    n231 = call "TriggerUpdate_Dynamic.vim"("Trigger"=w311) -> ("Update"=w310:bool)
    n232 = case shown="True" w310 {
      tunnel: w321 -> [_ w325]
      tunnel: w311 -> [_ w324]
      frame False {
      }
      frame True {
        n233 = call-poly <vilib>:"WPI_SolenoidSet.vi"("Value"=w324, "SolenoidDevRef"=w325) -> ()  [unwired: 8 in, 2 out]
      }
    }
    n234 = case shown="True" w308 {
      tunnel: w320 -> [_ w323]
      tunnel: w309 -> [_ w322]
      frame False {
      }
      frame True {
        n235 = call-poly <vilib>:"WPI_SolenoidSet.vi"("Value"=w322, "SolenoidDevRef"=w323) -> ()  [unwired: 8 in, 2 out]
      }
    }
    n236 = Wait (ms)(milliseconds to wait=u32 50) -> ()  [unwired: 1 out]
  }
  n237 = while {
    tunnel: w75 -> [w333]
    tunnel: w83 -> [_]
    stop <- FALSE stop-if-true
    n238 = global read "RobotStates.vi" "Upper Pulse State"() -> (w332:bool)
    n239 = Select(t=WPI_SolenoidValue."On" ("Value"), s=w332, f=WPI_SolenoidValue."Off") -> (s? t:f=w327:T23)
    n240 = call "TriggerUpdate_Dynamic.vim"("Trigger"=w327) -> ("Update"=w326:bool)
    n241 = case shown="True" w326 {
      tunnel: w333 -> [_ w335]
      tunnel: w327 -> [_ w334]
      frame False {
      }
      frame True {
        n242 = call-poly <vilib>:"WPI_SolenoidSet.vi"("Value"=w334, "SolenoidDevRef"=w335) -> ()  [unwired: 8 in, 2 out]
      }
    }
    n243 = Wait (ms)(milliseconds to wait=u32 50) -> ()  [unwired: 1 out]
  }
  n244 = global read "RefNums_Actuators.vi" "Drive_3L"() -> (w32:string)
  n245 = global read "RefNums_Actuators.vi" "Drive_1R"() -> (w28:string)
  n246 = global read "RefNums_Actuators.vi" "Drive_6R"() -> (w3:string)
  n247 = global read "RefNums_Actuators.vi" "Drive_5L"() -> (w4:string)
  n248 = global read "RefNums_Actuators.vi" "Drive_4L"() -> (w33:string)
  n249 = global read "RefNums_Actuators.vi" "Drive_2R"() -> (w29:string)
  n250 = call <vilib>:"WPI_MotorControlRefNum Registry Get.vi"("refnum name"=w3) -> ("MotorControlDevRef"=w1:T1)  [unwired: 9 in, 1 out]
  n251 = call <vilib>:"WPI_MotorControlRefNum Registry Get.vi"("refnum name"=w4) -> ("MotorControlDevRef"=w2:T1)  [unwired: 9 in, 1 out]
  n252 = call <vilib>:"WPI_MotorControlRefNum Registry Get.vi"("refnum name"=w33) -> ("MotorControlDevRef"=w24:T1)  [unwired: 9 in, 1 out]
  n253 = call <vilib>:"WPI_MotorControlRefNum Registry Get.vi"("refnum name"=w32) -> ("MotorControlDevRef"=w25:T1)  [unwired: 9 in, 1 out]
  n254 = call <vilib>:"WPI_MotorControlRefNum Registry Get.vi"("refnum name"=w29) -> ("MotorControlDevRef"=w26:T1)  [unwired: 9 in, 1 out]
  n255 = call <vilib>:"WPI_MotorControlRefNum Registry Get.vi"("refnum name"=w28) -> ("MotorControlDevRef"=w27:T1)  [unwired: 9 in, 1 out]
  n256 = while {
    shift-right: [w358] -> _
    shift-left: w83 -> [w358]
    shift-right: [w355] -> _
    shift-left: _ -> [w356]
    tunnel: w53 -> [w354]
    tunnel: [w346] -> _
    tunnel: w52 -> [w346]
    tunnel: w48 -> [w353]
    tunnel: w47 -> [w352]
    tunnel: w46 -> [w351]
    tunnel: w41 -> [w350]
    tunnel: w40 -> [w349]
    tunnel: w39 -> [w348]
    tunnel: w38 -> [w347]
    tunnel: w30 -> [w345]
    tunnel: w27 -> [w344]
    tunnel: w26 -> [w343]
    tunnel: w25 -> [w342]
    tunnel: w24 -> [w341]
    tunnel: w22 -> [w340]
    tunnel: w19 -> [w339]
    tunnel: w2 -> [w337]
    tunnel: w1 -> [w336]
    stop <- FALSE stop-if-true
    n257 = Tick Count (ms)() -> (millisecond timer value=w355:u32)
    n258 = Subtract(x=w355, y=w356) -> (x-y=→"Sensor Loop (ms)":u32)
    n259 = call "GetSensorValues.vi"("Ref_BuiltInAccelerometer"=w340, "Rear Prox Sensor"=w353, "Right Prox Sensor"=w352, "Left Prox Sensor"=w351, "Upper Pressure Transducer"=w350, "Ref_Compressor"=w346, "Front-Right Prox Sensor"=w349, "Ref_ElevatorEncoder"=w354, "Front-Left Prox Sensor"=w348, "Ref_ElevatorLimitSwitches"=w345, "Tank Pressure Transducer"=w347, "Ground Prox Sensor"=w339, "Ref_Drive 1R"=w344, "Ref_Drive 2R"=w343, "Ref_Drive 3L"=w342, "Ref_Drive 4L"=w341, "Ref_Drive 5L"=w337, "Ref_Drive 6R"=w336) -> ()  [unwired: 10 in]
    n260 = Wait (ms)(milliseconds to wait=u32 40) -> ()  [unwired: 1 out]
  }
